vi "Read Block.vi"(8 "error in (no error)":errorcluster, 11 "VisaComms in":refnum<class "VisaComms.lvclass">) -> (0 "error out":errorcluster, 2 "Block":string, 3 "VisaComms out":refnum<class "VisaComms.lvclass">, 5 "Buffer":string)   [LabVIEW 2020, in "CTI.lvlib" / "VisaComms.lvclass"]
uses:
  VisaComms.lvclass
  VisaComms.lvclass/VisaComms.ctl
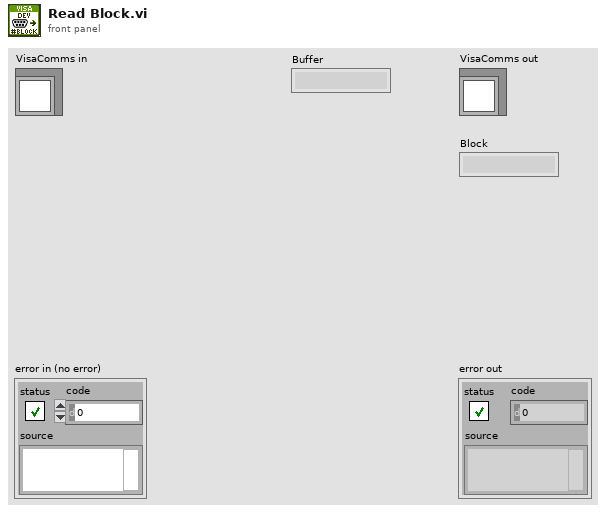
[diagram p1: front panel]
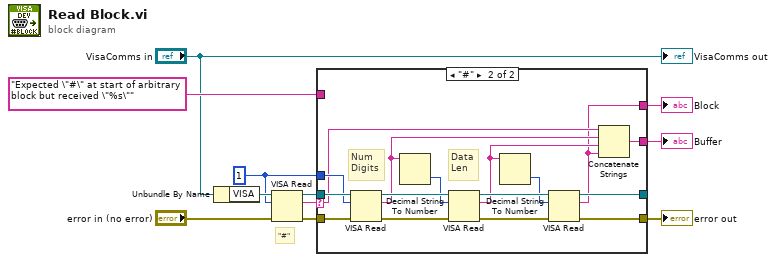
[diagram p0: block diagram]
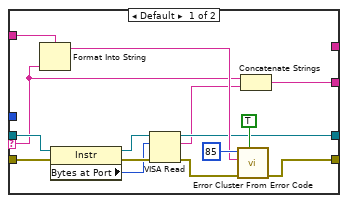
[diagram p2: hidden frame]
diagram:
  w2 = u32 1 ("byte count")
  # "\"#\""
  n1 = Unbundle By Name("VisaComms in") -> ("VISA"=w6:refnum<visa-resource-name>)
  n2 = VISA Read(VISA resource name=w6, byte count=w2, error in (no error)="error in (no error)") -> (VISA resource name out=w10:refnum<visa-resource-name>, read buffer=w11:string, error out=w9:errorcluster)  [unwired: 1 out]
  n3 = case shown="\"#\"" w11 {
    selector: w11 -> [w13 w31]
    tunnel: w10 -> [w20 w42]
    tunnel: w9 -> [w19 w41]
    tunnel: w2 -> [_ w40]
    tunnel: [w22 w32] -> w4
    tunnel: [w15 w33] -> _
    tunnel: [_ w28] -> w3
    tunnel: "Expected \"#\" at start of arbitrary block but received \"%s\"" -> [w21 _]
    tunnel: [w12 w27] -> w1
    frame Default {
      n4 = Format Into String(format string=w21, w13) -> (resulting string=w24:string)  [unwired: 2 in, 1 out]
      n5 = property class="Instr"(reference=w20, error in=w19) -> (reference out=w18:refnum<visa-resource-name>, error out=w26:errorcluster, "Bytes at Port"=w17:u32)
      n6 = VISA Read(VISA resource name=w18, byte count=w17, error in (no error)=w26) -> (VISA resource name out=w15:refnum<visa-resource-name>, read buffer=w14:string, error out=w16:errorcluster)  [unwired: 1 out]
      n7 = call <vilib>:"Error Cluster From Error Code.vi"("show call chain? (False)"=TRUE, "error in (no error)"=w16, "error message (\"\")"=w24, "error code (0)"=85) -> ("error out"=w22:errorcluster)  [unwired: 5 in]
      n8 = Concatenate Strings(w13, w14) -> (w12:string)
    }
    frame "#" {
      # "Data\nLen"
      # "Num\nDigits"
      n9 = VISA Read(VISA resource name=w42, byte count=w40, error in (no error)=w41) -> (VISA resource name out=w39:refnum<visa-resource-name>, read buffer=w30:string, error out=w38:errorcluster)  [unwired: 1 out]
      n10 = Decimal String To Number(string=w30) -> (number=w37:i32)  [unwired: 2 in, 1 out]
      n11 = VISA Read(VISA resource name=w39, byte count=w37, error in (no error)=w38) -> (VISA resource name out=w36:refnum<visa-resource-name>, read buffer=w29:string, error out=w35:errorcluster)  [unwired: 1 out]
      n12 = Decimal String To Number(string=w29) -> (number=w34:i32)  [unwired: 2 in, 1 out]
      n13 = VISA Read(VISA resource name=w36, byte count=w34, error in (no error)=w35) -> (VISA resource name out=w33:refnum<visa-resource-name>, read buffer=w28:string, error out=w32:errorcluster)  [unwired: 1 out]
      n14 = Concatenate Strings(w31, w30, w29, w28) -> (w27:string)
    }
  }
  "error out" <- w4
  "Block" <- w3
  "Buffer" <- w1
  "VisaComms out" <- "VisaComms in"
